vi "WebVideoGuide.vi"() -> ()   [LabVIEW 2021]
uses:
  <vilib>/sklein/WebView2/Webview2 Control/WebView2 Control.xctl
panel:
  out "WebView2 Control":string(xcontrol)
  in  "Msg":bool
  in  "Message to Page":string
  in  "Set JS 2":bool
  in  "Background":u32(colorbox)
  in  "stop":bool
  in  "Set JS":bool
  out "Message from Page":string
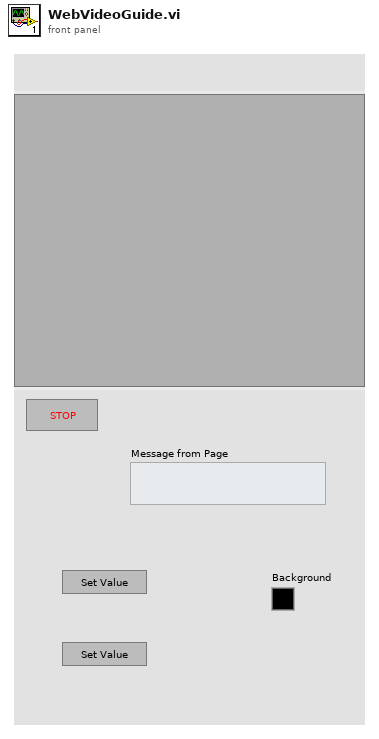
[diagram p1: front panel]
types:
  T1 = typedef "WebView2 Control.xctl/Events.ctl" = cluster{"Navigation Complete Event":refnum<user-event>, "Source Changed Event":refnum<user-event>, "Document Title Changed Event":refnum<user-event>, "Status Bar Text Changed":refnum<user-event>, "Web Message Received":refnum<user-event>, "Window Close Requested":refnum<user-event>, "DOM Loaded":refnum<user-event>, "Navigation Started Event":refnum<user-event>}
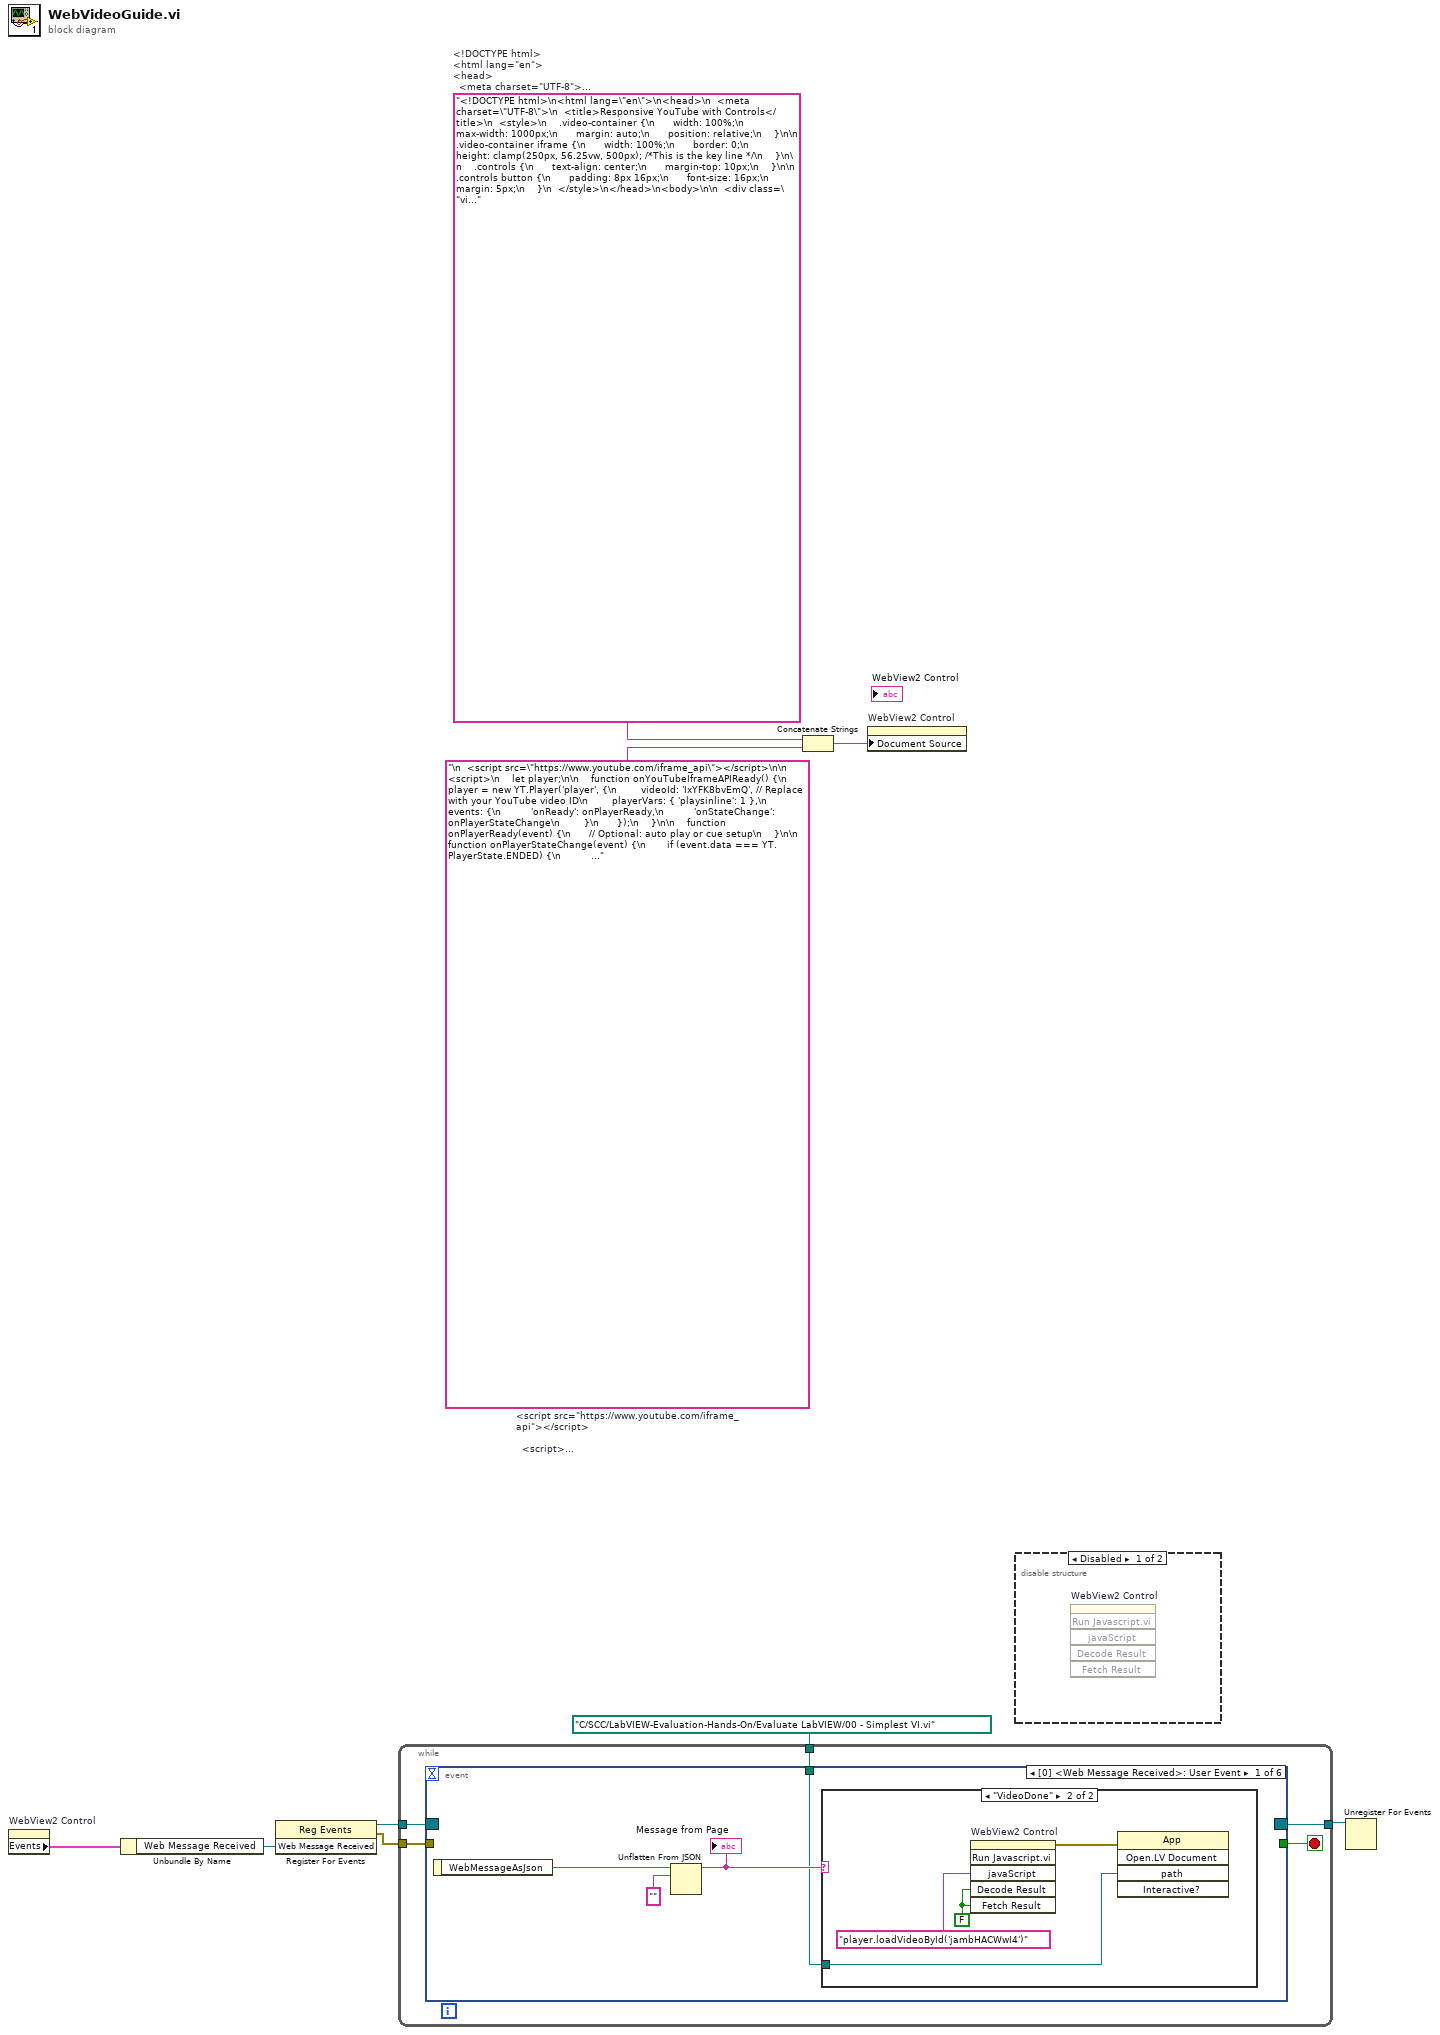
[diagram p0: block diagram]
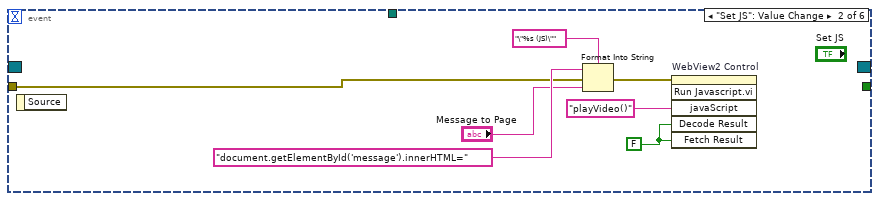
[diagram p4: hidden frame]
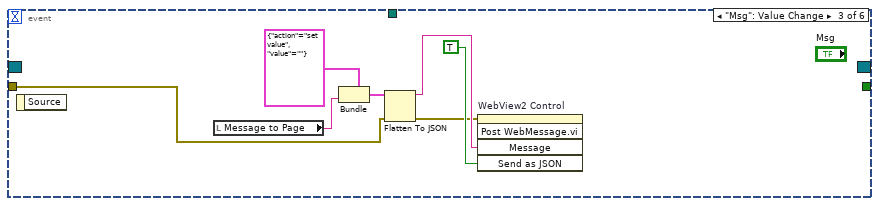
[diagram p5: hidden frame]
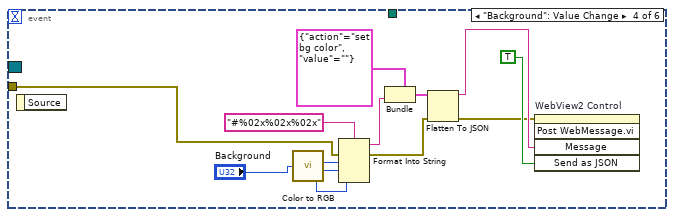
[diagram p6: hidden frame]
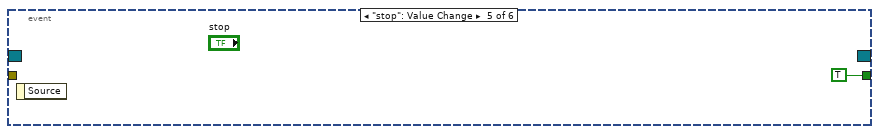
[diagram p7: hidden frame]
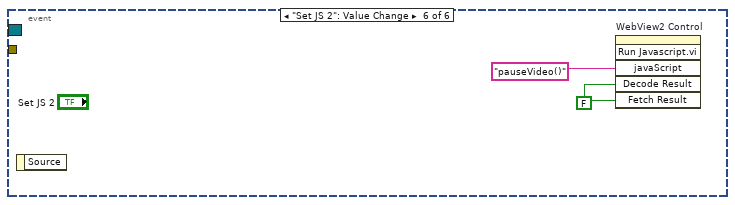
[diagram p8: hidden frame]
diagram:
  w1 = "<!DOCTYPE html>\n<html lang=\"en\">\n<head>\n  <meta charset=\"UTF-8\">\n  <title>Responsive YouTube with Controls</title>\n  <style>\n    .video-container {\n      width: 100%;\n      max-width: 1000px;\n      margin: auto;\n      position: relative;\n    }\n\n    .video-container iframe {\n      width: 100%;\n      border: 0;\n      height: clamp(250px, 56.25vw, 500px); /*This is the key line */\n    }\n\n    .controls {\n      text-align: center;\n      margin-top: 10px;\n    }\n\n    .controls button {\n      padding: 8px 16px;\n      font-size: 16px;\n      margin: 5px;\n    }\n  </style>\n</head>\n<body>\n\n  <div class=\"video-container\">\n    <div id=\"player\"></div>\n  </div>\n\n\n\n   \n"  # <!DOCTYPE html> <html lang="en"> <head>   <meta charset="UTF-8">   <title>Responsive YouTube with Controls</title>   <style>     .video-container {       width: 100%;       max-width: 1000px;       margin: auto;       position: relative;     }      .video-container iframe {       width: 100%;       border: 0;       height: clamp(250px, 56.25vw, 500px); /*This is the key line */     }      .controls {       text-align: center;       margin-top: 10px;     }      .controls button {       padding: 8px 16px;       font-size: 16px;       margin: 5px;     }   </style> </head> <body>    <div class="video-container">     <div id="player"></div>   </div>
  w4 = "\n  <script src=\"https://www.youtube.com/iframe_api\"></script>\n\n  <script>\n    let player;\n\n    function onYouTubeIframeAPIReady() {\n      player = new YT.Player('player', {\n        videoId: 'IxYFK8bvEmQ', // Replace with your YouTube video ID\n        playerVars: { 'playsinline': 1 },\n        events: {\n          'onReady': onPlayerReady,\n          'onStateChange': onPlayerStateChange\n        }\n      });\n    }\n\n    function onPlayerReady(event) {\n      // Optional: auto play or cue setup\n    }\n\n    function onPlayerStateChange(event) {\n       if (event.data === YT.PlayerState.ENDED) {\n            sendMessage()\n           } // Optional: auto play or cue setup\n    }\n\n\n    function playVideo() {\n      if (player) player.playVideo();\n    }\n\n    function pauseVideo() {\n      if (player) player.pauseVideo();\n    }\nfunction sendMessage() {\nwindow.chrome.webview.postMessage('VideoDone')\n}\n  </script>\n\n</body>\n</html>\n"  # <script src="https://www.youtube.com/iframe_api"></script>    <script>     let player;      function onYouTubeIframeAPIReady() {       player = new YT.Player('player', {         videoId: 'IxYFK8bvEmQ', // Replace with your YouTube video ID         playerVars: { 'playsinline': 1 },         events: {           'onReady': onPlayerReady,           'onStateChange': onPlayerStateChange         }       });     }      function onPlayerReady(event) {       // Optional: auto play or cue setup     }      function onPlayerStateChange(event) {        if (event.data === YT.PlayerState.ENDED) {             sendMessage()            } // Optional: auto play or cue setup     }       function playVideo() {       if (player) player.playVideo();     }      function pauseVideo() {       if (player) player.pauseVideo();     } function sendMessage() { window.chrome.webview.postMessage('VideoDone') }   </script>  </body> </html>
  n1 = property on="WebView2 Control" class="WebView2 Control (strict)"() -> ("Events"=w9:T1)  [unwired: 2 in, 2 out]
  n2 = Unbundle By Name(w9) -> ("Web Message Received"=w6:refnum<user-event>)
  n3 = register-events(w6) -> (reference out=w8:refnum<event-registration>, error out=w7:errorcluster)  [unwired: 2 in]
  n4 = while {
    tunnel: w8 -> [w12]
    tunnel: w7 -> [w13]
    tunnel: [w11] -> w5
    tunnel: path "C:/SCC/LabVIEW-Evaluation-Hands-On/Evaluate LabVIEW/00 - Simplest VI.vi" ("Path") -> [w10]
    stop <- w14 stop-if-true
    n5 = event shown="[0] <Web Message Received>: User Event" {
      selector: w12 -> [_ _ _ _ _ _]
      dyn-events: [_ _ _ _ _ _] -> w11
      timeout: _ -> [_ _ _ _ _ _]
      tunnel: [_ _ _ _ TRUE _] -> w14
      tunnel: w13 -> [_ w23 w31 w37 _ _]
      tunnel: w10 -> [w17 _ _ _ _ _]
      event User Event {
        n6 = event-data() -> ("WebMessageAsJson"=w15:string)  [unwired: 1 in]
        n7 = Unflatten From JSON(JSON string=w15, type and defaults="") -> (value=w18:string)  [unwired: 5 in, 1 out]
        "Message from Page" <- w18
        n8 = case shown="\"VideoDone\"" w18 {
          tunnel: w17 -> [_ w19]
          frame "False", Default {
          }
          frame "VideoDone" {
            w22 = FALSE ("Decode Result")
            n9 = invoke on="WebView2 Control" class="WebView2 Control (strict)" method="Run Javascript.vi"("javaScript"="player.loadVideoById('jambHACWwI4')", "Decode Result"=w22, "Fetch Result"=w22) -> (error out=w21:errorcluster)  [unwired: 3 in, 5 out]
            n10 = invoke class="App" method="Open.LV Document"(error in=w21, "path"=w19) -> ()  [unwired: 3 in, 5 out]
          }
        }
      }
      event "Set JS": Value Change {
        w25 = FALSE ("Fetch Result")
        n11 = event-data() -> ()  [unwired: 1 in, 1 out]
        n12 = Format Into String(format string="\"%s (JS)\"", initial string="document.getElementById('message').innerHTML=" ("javaScript"), error in=w23, "Message to Page") -> (error out=w26:errorcluster)  [unwired: 1 out]
        n13 = invoke on="WebView2 Control" class="WebView2 Control (strict)" method="Run Javascript.vi"(error in=w26, "javaScript"="playVideo()", "Decode Result"=w25, "Fetch Result"=w25) -> ()  [unwired: 2 in, 6 out]
      }
      event "Msg": Value Change {
        n14 = event-data() -> ()  [unwired: 1 in, 1 out]
        n15 = local read "Message to Page"() -> (w32:string)
        n16 = Bundle(cluster=cluster{"action":string, "value":string} {"action"="set value", "value"=""}, "value"=w32) -> (w35:cluster{"action":string, "value":string})  [unwired: 1 in]
        n17 = Flatten To JSON(anything=w35, error in (no error)=w31) -> (JSON string=w34:string, 11:w30:errorcluster)  [unwired: 1 in]
        n18 = invoke on="WebView2 Control" class="WebView2 Control (strict)" method="Post WebMessage.vi"(error in=w30, "Message"=w34, "Send as JSON"=TRUE) -> ()  [unwired: 2 in, 5 out]
      }
      event "Background": Value Change {
        n19 = event-data() -> ()  [unwired: 1 in, 1 out]
        n20 = call <vilib>:"Color to RGB.vi"("Color"="Background") -> ("R"=w41:u8, "G"=w40:u8, "B"=w39:u8)  [unwired: 1 out]
        n21 = Format Into String(format string="#%02x%02x%02x", error in=w37, w41, w40, w39) -> (resulting string=w44:string, error out=w43:errorcluster)  [unwired: 1 in]
        n22 = Bundle(cluster=cluster{"action":string, "value":string} {"action"="set bg color", "value"=""}, "value"=w44) -> (w48:cluster{"action":string, "value":string})  [unwired: 1 in]
        n23 = Flatten To JSON(anything=w48, error in (no error)=w43) -> (JSON string=w47:string, 11:w38:errorcluster)  [unwired: 1 in]
        n24 = invoke on="WebView2 Control" class="WebView2 Control (strict)" method="Post WebMessage.vi"(error in=w38, "Message"=w47, "Send as JSON"=TRUE) -> ()  [unwired: 2 in, 5 out]
      }
      event "stop": Value Change {
        n25 = event-data() -> ()  [unwired: 1 in, 1 out]
      }
      event "Set JS 2": Value Change {
        w51 = FALSE ("Decode Result")
        n26 = event-data() -> ()  [unwired: 1 in, 1 out]
        n27 = invoke on="WebView2 Control" class="WebView2 Control (strict)" method="Run Javascript.vi"("javaScript"="pauseVideo()", "Decode Result"=w51, "Fetch Result"=w51) -> ()  [unwired: 3 in, 6 out]
      }
    }
  }
  n28 = Concatenate Strings(w1, w4) -> (w3:string)
  n29 = property on="WebView2 Control" class="WebView2 Control (strict)"("Document Source"=w3) -> ()  [unwired: 2 in, 2 out]
  n30 = disable-structure shown="Disabled" {
    frame Disabled {
      n31 = invoke on="WebView2 Control" class="WebView2 Control (strict)" method="Run Javascript.vi"() -> ()  [unwired: 6 in, 6 out]
    }
    frame Enabled {
    }
  }
  n32 = Unregister For Events(event registration refnum=w5) -> ()  [unwired: 1 in, 1 out]
